vi "通用参数设置.vi"(11 "通用寄存器配置输入":T1) -> (3 "通用寄存器配置输出":u32[](array[numeric]))   [LabVIEW 2012]
uses:
  u16-u8s.vi
  u32-u8s.vi
panel:
  out "添加的数组":u8[](array[numeric])
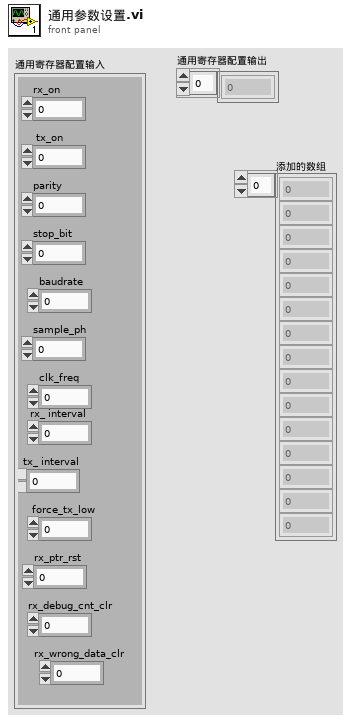
[diagram p1: front panel]
types:
  T1 = cluster{"rx_on":u8, " tx_on":u8, "parity":u8, "stop_bit":u8, "baudrate":u16, "sample_ph":u16, "clk_freq":u32, "rx_ interval":u16, "tx_ interval":u16, "force_tx_low":u32, "rx_ptr_rst":u8, "rx_debug_cnt_clr":u8, "rx_wrong_data_clr":u16}
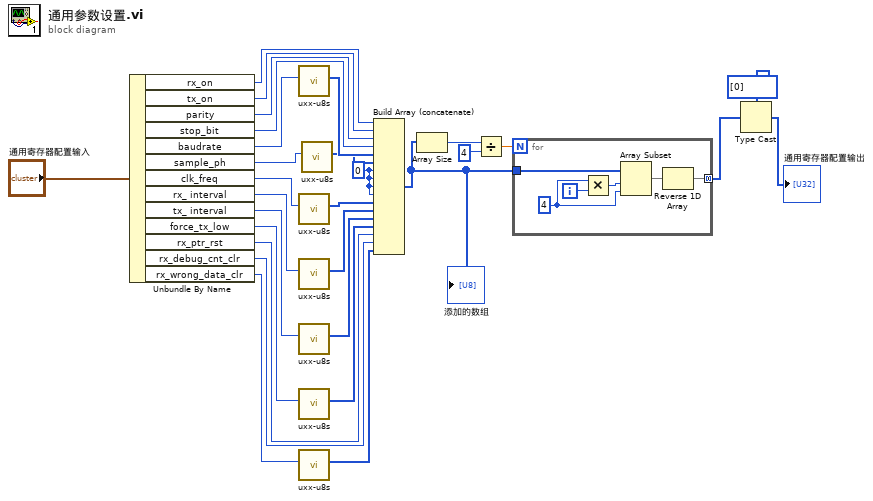
[diagram p0: block diagram]
diagram:
  w5 = u8 0 ("元素")
  n1 = Unbundle By Name("通用寄存器配置输入") -> ("rx_on"=w25:u8, "tx_on"=w26:u8, "parity"=w27:u8, "stop_bit"=w20:u8, "baudrate"=w19:u16, "sample_ph"=w7:u16, "clk_freq"=w17:u32, "rx_ interval"=w15:u16, "tx_ interval"=w13:u16, "force_tx_low"=w11:u32, "rx_ptr_rst"=w28:u8, "rx_debug_cnt_clr"=w29:u8, "rx_wrong_data_clr"=w9:u16)
  n2 = call-poly "uxx-u8s.vi"("数值"=w19) -> ("反转的数组"=w18:u8[])  [unwired: 10 in]
  n3 = call-poly "uxx-u8s.vi"("数值"=w17) -> ("反转的数组"=w16:u8[])  [unwired: 10 in]
  n4 = call-poly "uxx-u8s.vi"("数值"=w15) -> ("反转的数组"=w14:u8[])  [unwired: 10 in]
  n5 = call-poly "uxx-u8s.vi"("数值"=w13) -> ("反转的数组"=w12:u8[])  [unwired: 10 in]
  n6 = call-poly "uxx-u8s.vi"("数值"=w11) -> ("反转的数组"=w10:u8[])  [unwired: 10 in]
  n7 = call-poly "uxx-u8s.vi"("数值"=w9) -> ("反转的数组"=w8:u8[])  [unwired: 10 in]
  n8 = call-poly "uxx-u8s.vi"("数值"=w7) -> ("反转的数组"=w6:u8[])  [unwired: 10 in]
  n9 = Build Array (concatenate)(w25, w26, w27, w20, w18, w6, w5, w5, w5, w5, w16, w14, w12, w10, w28, w29, w8) -> (w4:u8[])
  "添加的数组" <- w4
  n10 = Array Size(array=w4) -> (size(s)=w23:i32)
  n11 = Divide(x=w23, y=4) -> (x/y=w21:dbl)
  n12 = for {
    N: w21 -> [_]
    tunnel: w4 -> [w35]
    tunnel: [w30] -> w2 mode=concatenating
    i -> [w34]
    w32 = 4 ("x")
    n13 = Multiply(x=w32, y=w34) -> (x*y=w33:i32)
    n14 = Array Subset(array=w35, index=w33, length=w32) -> (w31:u8[])
    n15 = Reverse 1D Array(array=w31) -> (reversed array=w30:u8[])
  }
  n16 = Type Cast(type=u32[] [0], x=w2) -> (*(type *) &x=→"通用寄存器配置输出":u32[])
